vi "Return Parameter Status.vi"(4 "error":string, 6 "Status":T1, 8 "error in (no error)":errorcluster, 9 "Parameter Name":string, 10 "IED Name":string, 11 "SCADA in":refnum<class "SCADA.lvclass">) -> (0 "error out":errorcluster, 3 "SCADA out":refnum<class "SCADA.lvclass">)   [LabVIEW 2015, in "SCADA Core.lvlib" / "SCADA.lvclass"]
uses:
  SCADA.lvclass
  SCADA Abstract Messages/Set Device Parameter Status Msg/Set Device Parameter Status.ctl
  <vilib>/ActorFramework/Actor/Actor.lvclass/Actor.ctl
  SCADA.lvclass/SCADA.ctl
  SCADA Abstract Messages/Set Device Parameter Status Msg/Set Device Parameter Status Msg.lvclass
  <vilib>/ActorFramework/Actor/Actor.lvclass
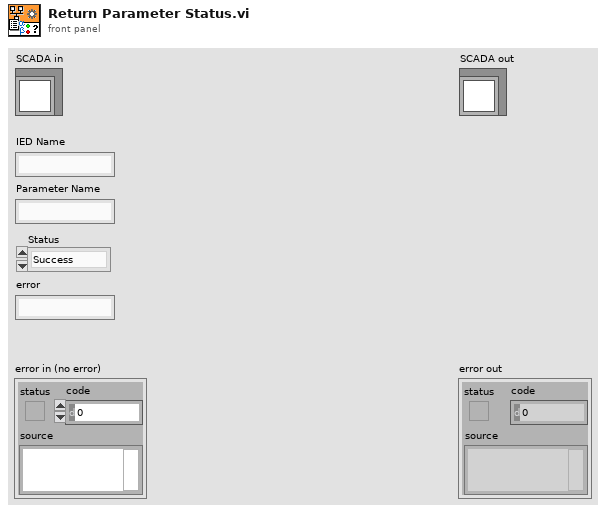
[diagram p1: front panel]
types:
  T1 = typedef "SCADA Core.lvlib/Set Device Parameter Status Msg.lvclass/Set Device Parameter Status.ctl" = enum16{"Success", "Failure"}
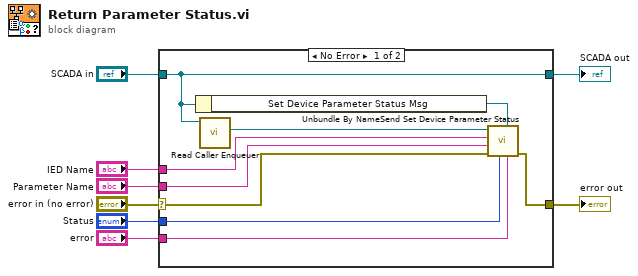
[diagram p0: block diagram]
diagram:
  n1 = case shown="No Error" "error in (no error)" {
    selector: "error in (no error)" -> [w14 w19]
    tunnel: [w13 w19] -> w7
    tunnel: [w17 w18] -> w5
    tunnel: "SCADA in" -> [w17 w18]
    tunnel: "IED Name" -> [w12 _]
    tunnel: "Parameter Name" -> [w11 _]
    tunnel: "Status" -> [w10 _]
    tunnel: "error" -> [w9 _]
    frame No Error {
      n2 = Unbundle By Name(w17) -> ("Set Device Parameter Status Msg"=w15:refnum<class "Set Device Parameter Status Msg.lvclass">)
      n3 = call <vilib>:"Read Caller Enqueuer.vi"("Actor"=w17) -> ("Caller Enqueuer"=w16:refnum<class "Message Enqueuer.lvclass">)  [unwired: 10 in]
      n4 = call "Send Set Device Parameter Status.vi"("error string"=w9, "Set Device Parameter Status Msg"=w15, "Status"=w10, "error in (no error)"=w14, "Parameter Name"=w11, "IED Name"=w12, "Message Enqueuer in"=w16) -> ("error out"=w13:errorcluster)  [unwired: 3 in, 1 out]
    }
    frame Error {
    }
  }
  "error out" <- w7
  "SCADA out" <- w5
